vi "Graph1.vi"(6 "Массив точек":dbl[](array[numeric]), 9 "Частота (1000 Hz)":dbl, 10 "Количество точек":dbl, 11 "Амплитуда оси Y":dbl) -> (2 "График":cluster{"Y":dbl[], "Y":dbl[]}[](graph) caption="XY Graph 3")   [LabVIEW 2012]
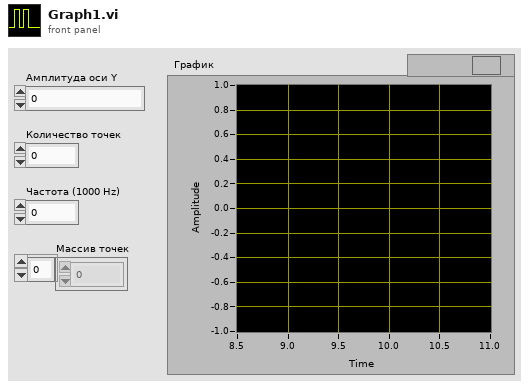
[diagram p1: front panel]
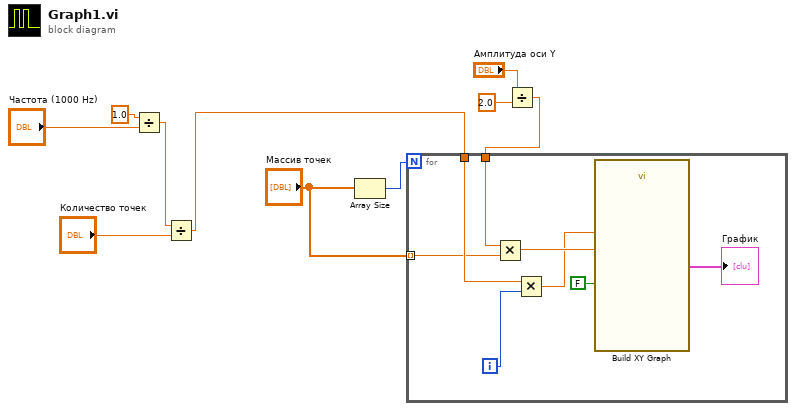
[diagram p0: block diagram]
diagram:
  n1 = Divide(x=1.0, y="Частота (1000 Hz)") -> (x/y=w7:dbl)
  n2 = Divide(x=w7, y="Количество точек") -> (x/y=w8:dbl)
  n3 = Array Size(array="Массив точек") -> (size(s)=w5:i32)
  n4 = Divide(x="Амплитуда оси Y", y=2.0) -> (x/y=w1:dbl)
  n5 = for {
    N: w5 -> [_]
    tunnel: "Массив точек" -> [w13] mode=indexing
    tunnel: w1 -> [w12]
    tunnel: w8 -> [w15]
    i -> [w14]
    n6 = Multiply(x=w12, y=w13) -> (x*y=w17:dbl)
    n7 = Multiply(x=w15, y=w14) -> (x*y=w16:dbl)
    n8 = call "Build XY Graph"("Reset"=FALSE, "Y Input"=w17, "X Input"=w16) -> ("XY Graph"=→"График":cluster{"Y":dbl[], "Y":dbl[]}[])  [unwired: 2 in, 6 out]
  }
